vi "weights_biases_import_sub.vi"(2 "format (%.3f)":string="%.3f", 3 "Import_biases_cvs":path=path "C:/Users/HYPC/Desktop/WB/biases_0.csv", 4 "Import_weights_cvs":path=path "C:/Users/HYPC/Desktop/WB/weights_0.csv") -> (0 "biases_1d":dbl[](array[numeric]), 1 "weigths_2D":dbl[][](array[numeric]))   [LabVIEW 2021]
uses:
  <vilib>/Utility/file.llb/Read Delimited Spreadsheet (DBL).vi
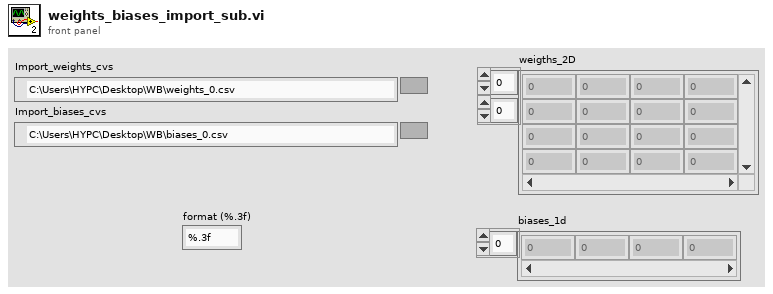
[diagram p1: front panel]
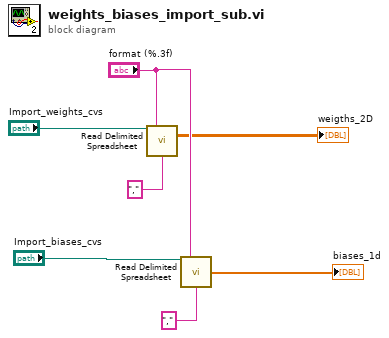
[diagram p0: block diagram]
diagram:
  n1 = call-poly <vilib>:"Read Delimited Spreadsheet.vi"("file path (dialog if empty)"="Import_weights_cvs", "format (%.3f)"="format (%.3f)", "delimiter (\\t)"="," ("delimiter (\\t)")) -> ("all rows"=→"weigths_2D":dbl[][])  [unwired: 7 in, 5 out]
  n2 = call-poly <vilib>:"Read Delimited Spreadsheet.vi"("file path (dialog if empty)"="Import_biases_cvs", "format (%.3f)"="format (%.3f)", "delimiter (\\t)"="," ("delimiter (\\t)")) -> ("first row"=→"biases_1d":dbl[])  [unwired: 7 in, 5 out]
